vi "Read Current champion_.vi"(8 "error in (no error)":errorcluster, 11 "WWF Wrestler in":refnum<class "WWE Wrestler.lvclass">) -> (0 "error out":errorcluster, 2 "Current champion?":bool, 3 "WWF Wrestler out":refnum<class "WWE Wrestler.lvclass">)   [LabVIEW 2019, in "WWE Wrestler.lvclass"]
uses:
  WWE Wrestler.lvclass
  WWE Wrestler.lvclass/WWE Wrestler.ctl
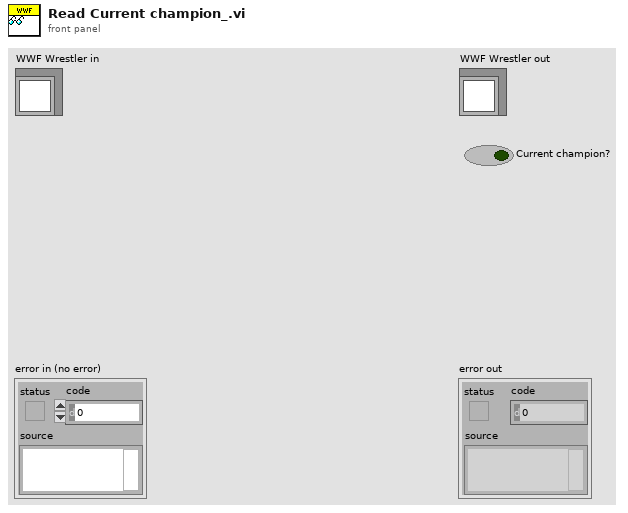
[diagram p1: front panel]
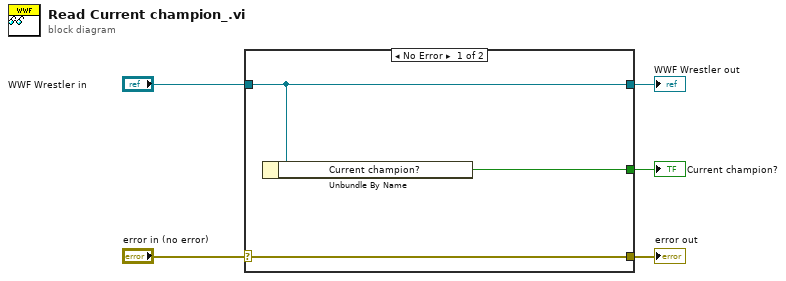
[diagram p0: block diagram]
diagram:
  n1 = case shown="No Error" "error in (no error)" {
    selector: "error in (no error)" -> [w8 w9]
    tunnel: [w8 w9] -> w4
    tunnel: [w7 w10] -> w2
    tunnel: "WWF Wrestler in" -> [w7 w10]
    tunnel: [w6 _] -> w1
    frame No Error {
      n2 = Unbundle By Name(w7) -> ("Current champion?"=w6:bool)
    }
    frame Error {
    }
  }
  "error out" <- w4
  "WWF Wrestler out" <- w2
  "Current champion?" <- w1
